vi "Is File.vi"(1 "Input Path":path) -> (0 "Is Existing File?":bool)   [LabVIEW 2023, in "Error Manager.lvlib"]
uses:
  Error Manager.lvlib
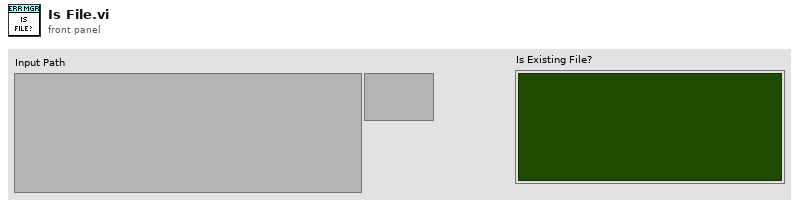
[diagram p1: front panel]
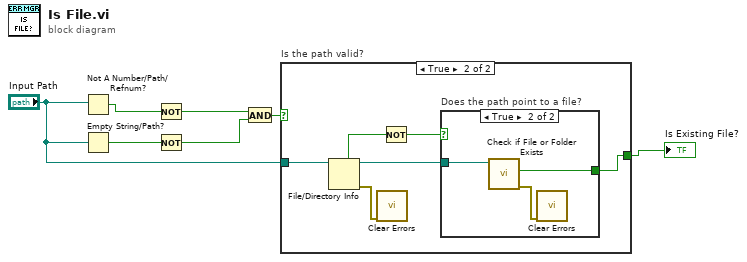
[diagram p0: block diagram]
diagram:
  n1 = Not A Number/Path/Refnum?(number/path/refnum="Input Path") -> (NaN/Path/Refnum?=w5:bool)
  n2 = Empty String/Path?(string/path="Input Path") -> (empty?=w6:bool)
  n3 = Not(x=w5) -> (.not. x?=w2:bool)
  n4 = Not(x=w6) -> (.not. x?=w1:bool)
  n5 = And(x=w2, y=w1) -> (x .and. y?=w3:bool)
  n6 = case "Is the path valid?" shown="True" w3 {
    tunnel: [_ w9] -> w7
    tunnel: "Input Path" -> [_ w13]
    frame False {
    }
    frame True {
      n7 = File/Directory Info(path=w13) -> (path out=w10:path, directory=w12:bool, error out=w8:errorcluster)  [unwired: 1 in, 4 out]
      n8 = call <vilib>:"Clear Errors.vi"("error in (no error)"=w8) -> ()  [unwired: 5 in, 2 out]
      n9 = Not(x=w12) -> (.not. x?=w11:bool)
      n10 = case "Does the path point to a file?" shown="True" w11 {
        tunnel: w10 -> [_ w16]
        tunnel: [_ w15] -> w9
        frame False {
        }
        frame True {
          n11 = call <vilib>:"Check if File or Folder Exists.vi"("path"=w16) -> ("error out"=w14:errorcluster, "file or folder exists?"=w15:bool)  [unwired: 8 in, 1 out]
          n12 = call <vilib>:"Clear Errors.vi"("error in (no error)"=w14) -> ()  [unwired: 5 in, 2 out]
        }
      }
    }
  }
  "Is Existing File?" <- w7
